vi "SPCFormatError_HH.vi"(1 "Error Code":i32, 2 "Source":string) -> (0 "error out":errorcluster)   [LabVIEW 2009]
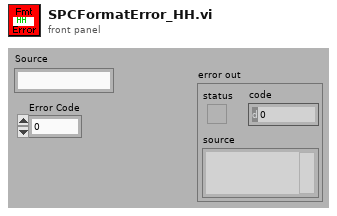
[diagram p1: front panel]
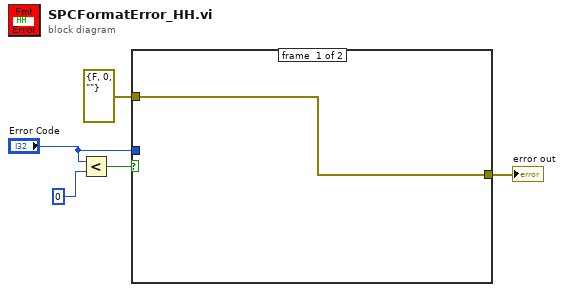
[diagram p0: block diagram]
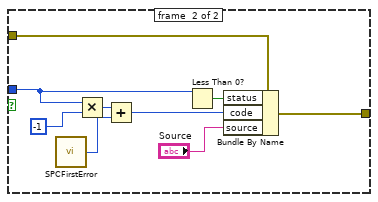
[diagram p2: hidden frame]
diagram:
  n1 = Less?(x="Error Code", y=0) -> (x < y?=w3:bool)
  n2 = case shown="True" w3 {
    tunnel: "Error Code" -> [_ w8]
    tunnel: errorcluster {"status"=FALSE, "code"=0, "source"=""} ("error out") -> [w6 w12]
    tunnel: [w6 w7] -> w1
    frame #0 {
    }
    frame #1 {
      n3 = call "SPCFirstError.vi"() -> ("First Error (output)"=w13:i32)  [unwired: 2 in]
      n4 = Multiply(x=w8, y=-1) -> (x*y=w14:i32)
      n5 = Add(x=w14, y=w13) -> (x+y=w11:i32)
      n6 = Less Than 0?(x=w8) -> (x < 0?=w9:bool)
      n7 = Bundle By Name(cluster=w12, "status"=w9, "code"=w11, "source"="Source") -> (w7:errorcluster)
    }
  }
  "error out" <- w1
